vi "populateTelemetryHardpointData.vi"(8 "error in (no error)":errorcluster, 11 "Model in":refnum<class "Model.lvclass">) -> (0 "error out":errorcluster, 3 "Model out":refnum<class "Model.lvclass">)   [LabVIEW 2016, in "Model.lvclass"]
uses:
  Model.lvclass
  Model.lvclass/Model.ctl
  ILCCommunications/ILCCommunications.lvclass/ILCCommunications.ctl
  Publisher/Publisher.lvclass/Publisher.ctl
  Common_RT_HPILC/HPILC/HPILC.lvclass/HPILC.ctl
  ILCCommunications/ILCCommunications.lvclass
  Common_RT_HPILC/HPILC/HPILC.lvclass
  Publisher/Publisher.lvclass
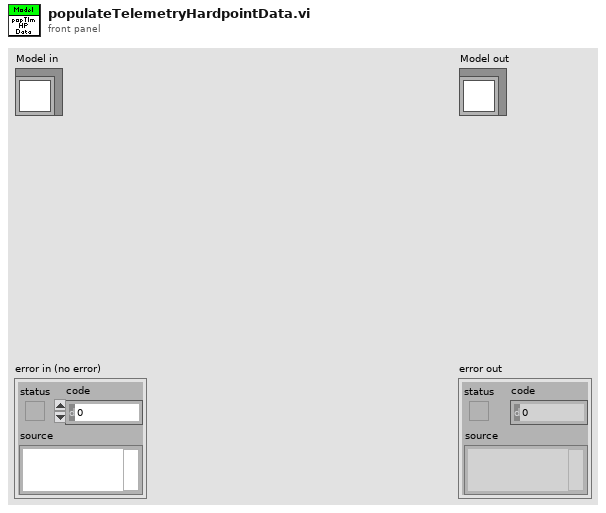
[diagram p1: front panel]
types:
  T1 = typedef "M1M3SupportTopics.lvlib/Timestamp.ctl" = dbl
  T2 = typedef "RTHPILC.lvlib/HPData.ctl" = cluster{"Constants":T3, "Command":T4, "Telemetry":T5, "Responses":T6, "Timings":T8, "Timestamps":T9}
  T3 = typedef "RTHPILC.lvlib/HPConstants.ctl" = cluster{"ID":i16, "ReferencePosition":i32, "XPosition":sgl, "YPosition":sgl, "ZPosition":sgl}
  T4 = typedef "RTHPILC.lvlib/HPCommand.ctl" = cluster{"Steps":i8}
  T5 = typedef "RTHPILC.lvlib/HPTelemetry.ctl" = cluster{"ILCFault":bool, "LimitSwitchCWOperated":bool, "LimitSwitchCCWOperated":bool, "BroadcastCounter":u8, "SSIEncoderValue":i32, "LoadCellForce":sgl}
  T6 = typedef "RTHPILC.lvlib/HPResponses.ctl" = cluster{"StepMotor":T7, "ForceAndStatus":T7}
  T7 = typedef "RTModbus.lvlib/ExceptionCodes.ctl" = u16
  T8 = typedef "RTHPILC.lvlib/HPTimings.ctl" = cluster{"BroadcastStepMotor":u32, "ForceAndStatus":u32, "FreezeSensorValues":u32, "StepMotor":u32}
  T9 = typedef "RTHPILC.lvlib/HPTimestamps.ctl" = cluster{"StepMotor":dbl, "ForceAndStatus":dbl}
  T10 = typedef "M1M3SupportTopics.lvlib/TelemetryHardpointData.ctl" = cluster{"Timestamp":T1, "StepsCommanded":i16[], "Force":sgl[], "Encoder":i32[], "ILCFault":bool[], "CWLimitOperated":bool[], "CCWLimitOperated":bool[], "BroadcastCounter":u8[]}
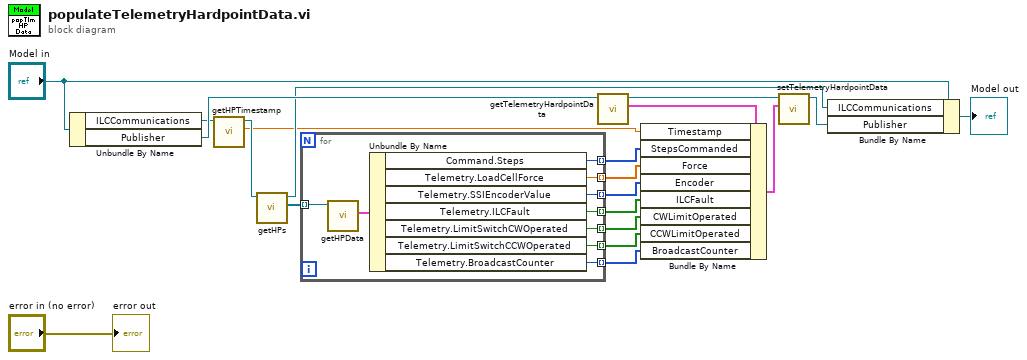
[diagram p0: block diagram]
diagram:
  n1 = Unbundle By Name("Model in") -> ("ILCCommunications"=w4:refnum<class "ILCCommunications.lvclass">, "Publisher"=w19:refnum<class "Publisher.lvclass">)
  n2 = call "getHPTimestamp.vi"("ILCCommunications in"=w4) -> ("Timestamp"=w2:T1, "ILCCommunications out"=w3:refnum<class "ILCCommunications.lvclass">)  [unwired: 9 in]
  n3 = call "getHPs.vi"("ILCCommunications in"=w3) -> ("HPs"=w16:refnum<class "HPILC.lvclass">[], "ILCCommunications out"=w5:refnum<class "ILCCommunications.lvclass">)  [unwired: 9 in]
  n4 = for {
    tunnel: w16 -> [w29] mode=indexing
    tunnel: [w27] -> w7 mode=indexing
    tunnel: [w26] -> w9 mode=indexing
    tunnel: [w25] -> w10 mode=indexing
    tunnel: [w24] -> w11 mode=indexing
    tunnel: [w23] -> w8 mode=indexing
    tunnel: [w22] -> w13 mode=indexing
    tunnel: [w21] -> w12 mode=indexing
    n5 = call "getHPData.vi"("HPILC in"=w29) -> ("HPData"=w28:T2)  [unwired: 9 in, 1 out]
    n6 = Unbundle By Name(w28) -> ("Command.Steps"=w27:i8, "Telemetry.LoadCellForce"=w23:sgl, "Telemetry.SSIEncoderValue"=w26:i32, "Telemetry.ILCFault"=w25:bool, "Telemetry.LimitSwitchCWOperated"=w24:bool, "Telemetry.LimitSwitchCCWOperated"=w22:bool, "Telemetry.BroadcastCounter"=w21:u8)
  }
  n7 = call "getTelemetryHardpointData.vi"("Publisher in"=w19) -> ("TelemetryHardpointData"=w18:T10, "Publisher out"=w17:refnum<class "Publisher.lvclass">)  [unwired: 9 in]
  n8 = Bundle By Name(cluster=w18, "Timestamp"=w2, "StepsCommanded"=w7, "Force"=w8, "Encoder"=w9, "ILCFault"=w10, "CWLimitOperated"=w11, "CCWLimitOperated"=w13, "BroadcastCounter"=w12) -> (w6:T10)
  n9 = call "setTelemetryHardpointData.vi"("TelemetryHardpointData"=w6, "Publisher in"=w17) -> ("Publisher out"=w15:refnum<class "Publisher.lvclass">)  [unwired: 9 in]
  n10 = Bundle By Name(cluster="Model in", "ILCCommunications"=w5, "Publisher"=w15) -> (→"Model out":refnum<class "Model.lvclass">)
  "error out" <- "error in (no error)"
